vi "AB_820_850_Project_DestinationItems.vi"(6 "usedDestinations":i32[](array[numeric]), 7 "action":T3, 8 "error in (no error)":errorcluster, 9 "buildType":T1, 10 "oldBuildObject":T2, 11 "buildObject":T2) -> (0 "error out":errorcluster, 3 "buildObject out":T2)   [LabVIEW 2020]
doc: "Reads and writes the data to the object property bag."
uses:
  <resource>/Framework/Providers/API/ItemRef.ctl
  <vilib>/AppBuilder/RW_Project/AB_RW_Project_PropBag_ArrayAction.ctl
  <vilib>/AppBuilder/AB_BuildType.ctl
  <vilib>/AppBuilder/RW_Project/AB_RW_Project_PropBag_Action.ctl
  <resource>/Framework/Providers/Common/provcom_StringGlobals.vi
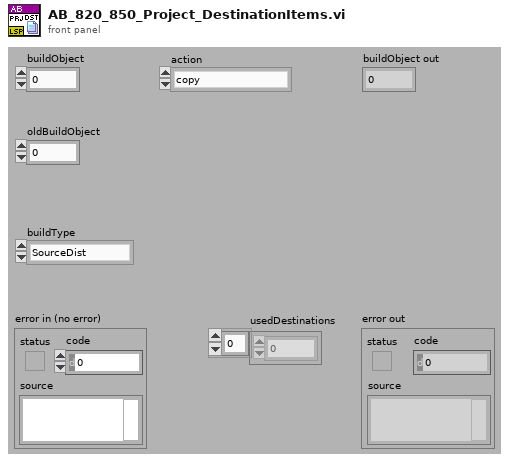
[diagram p1: front panel]
types:
  T1 = typedef "AB_BuildType.ctl" = enum16{"SourceDist", "EXE", "DLL", "RTExe"}
  T2 = typedef "ItemRef.ctl" = u64
  T3 = typedef "AB_RW_Project_PropBag_ArrayAction.ctl" = enum16{"copy", "saveForPrevious", "loadFromPrevious", "clear"}
  T4 = typedef "AB_RW_Project_PropBag_Action.ctl" = enum16{"read", "write", "clear", "readPrevious", "writePrevious", "clearPrevious"}
  T5 = cluster{"destName":string, "path":path, "preserveHierarchy":bool, "libraryName":string}
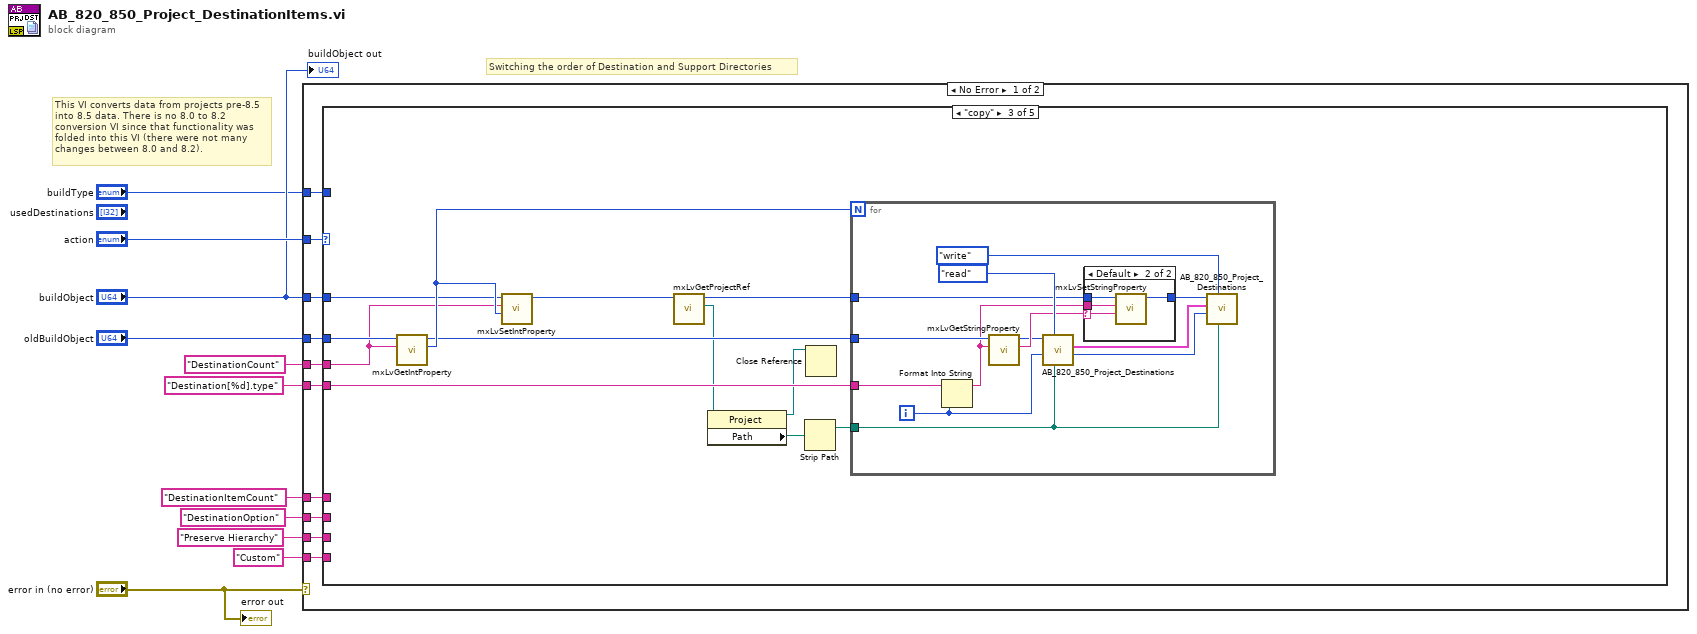
[diagram p0: block diagram]
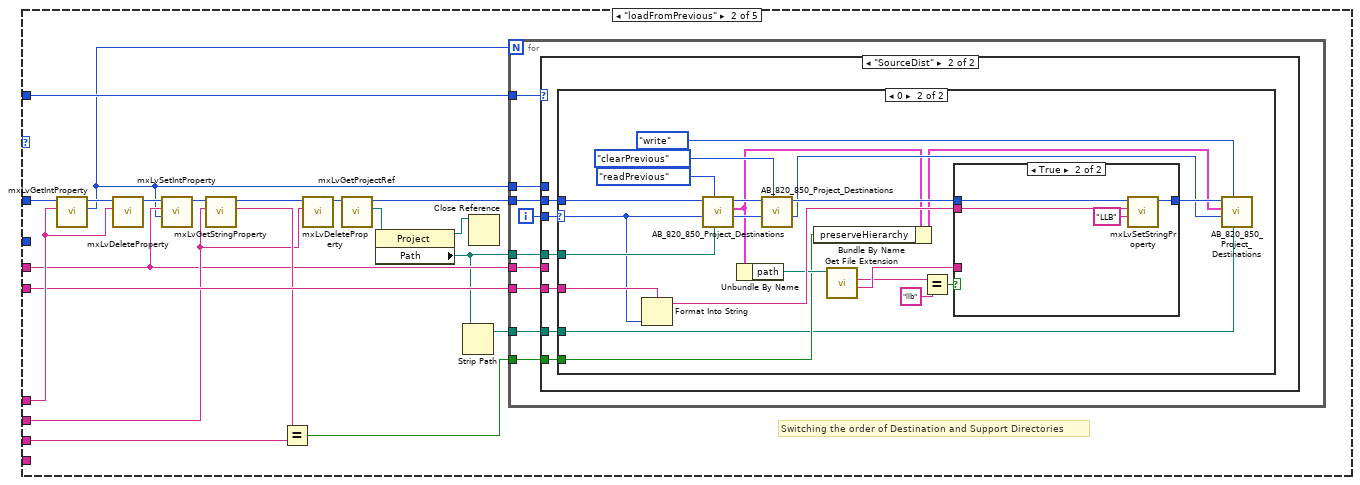
[diagram p3: hidden frame]
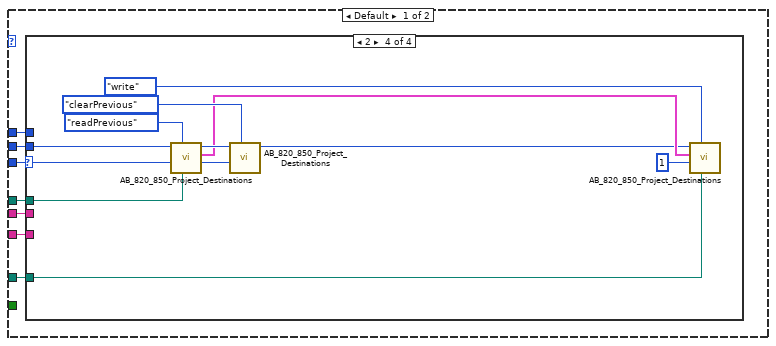
[diagram p4: hidden frame]
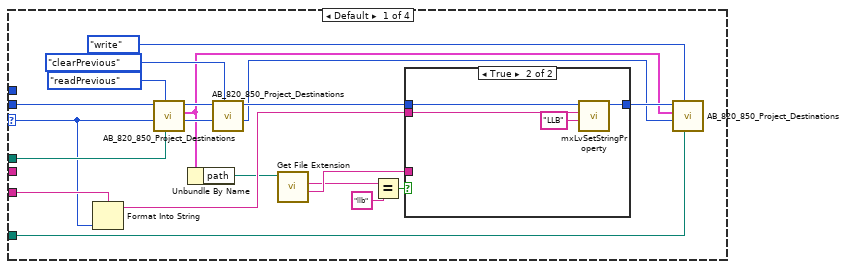
[diagram p5: hidden frame]
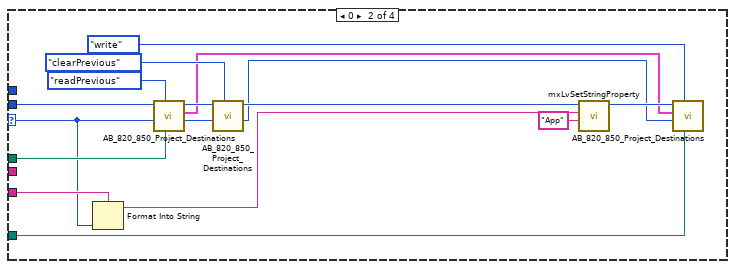
[diagram p7: hidden frame]
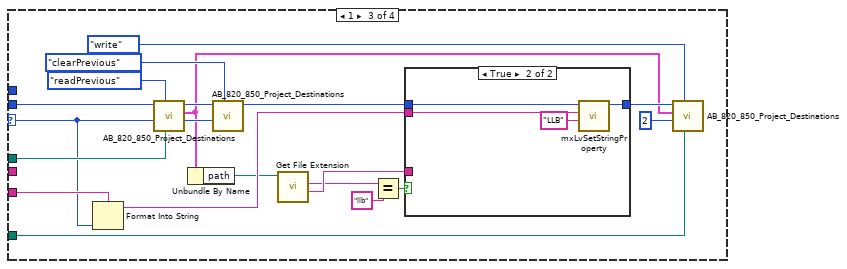
[diagram p8: hidden frame]
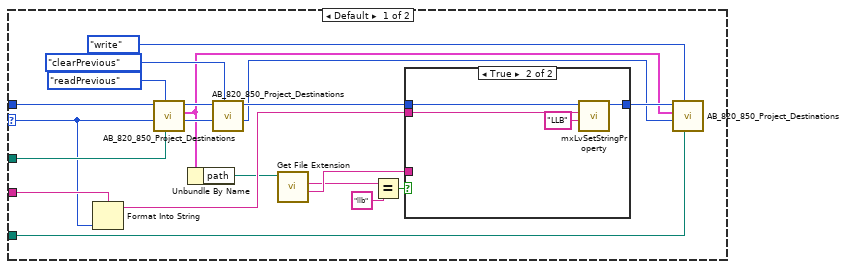
[diagram p10: hidden frame]
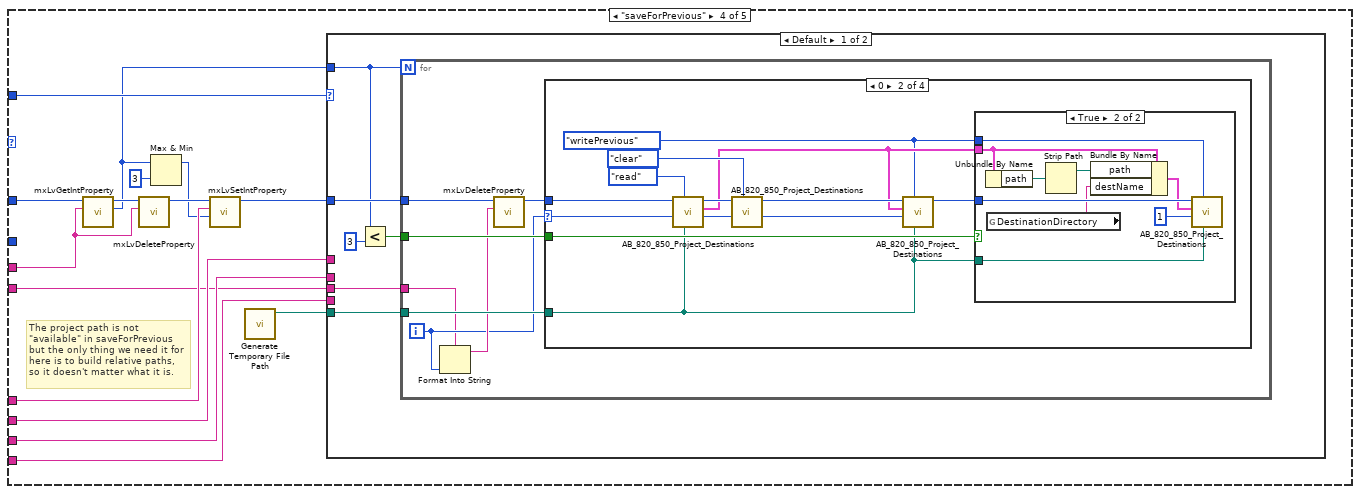
[diagram p14: hidden frame]
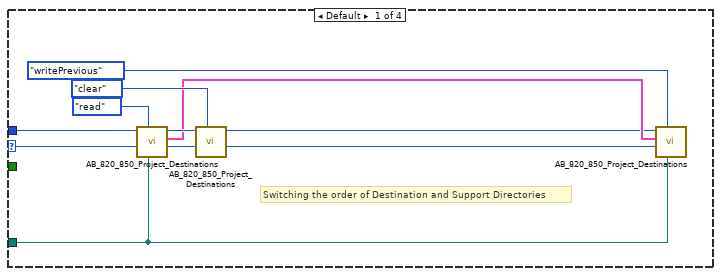
[diagram p15: hidden frame]
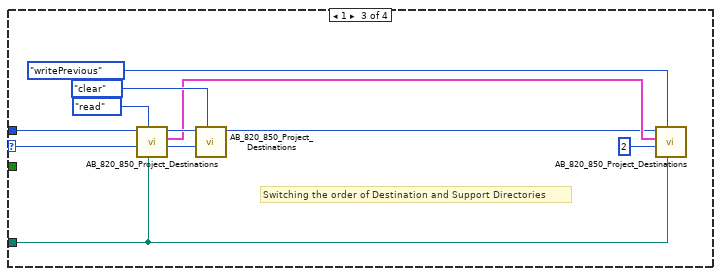
[diagram p17: hidden frame]
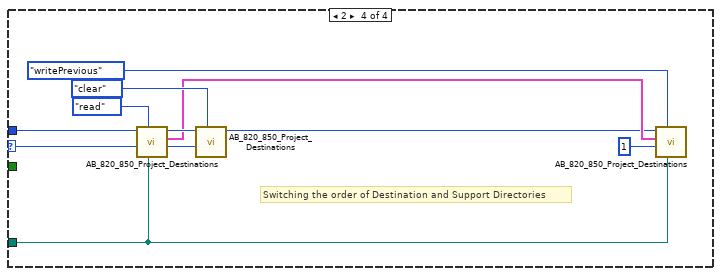
[diagram p18: hidden frame]
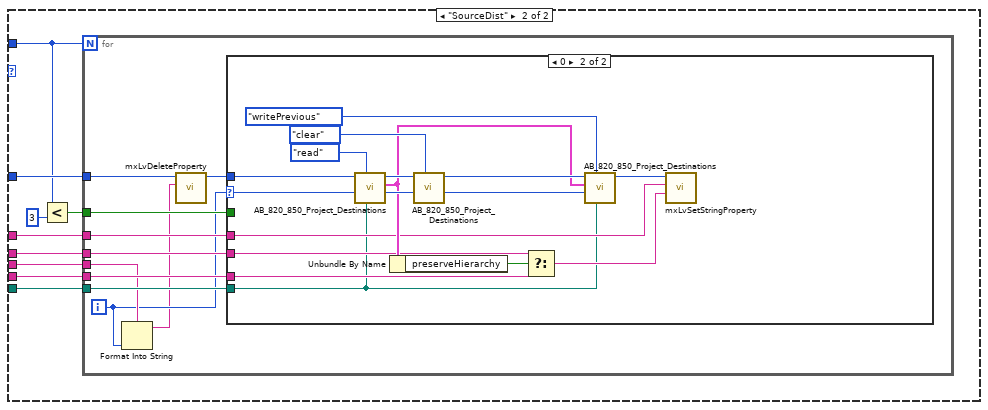
[diagram p19: hidden frame]
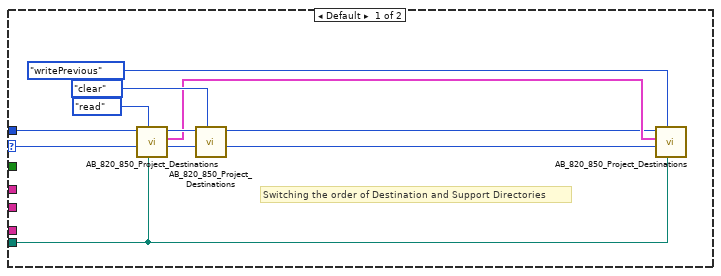
[diagram p20: hidden frame]
diagram:
  # "This VI converts data from projects pre-8.5 into 8.5 data. There is no 8.0 to 8.2 conversion VI since that functionality was folded into this VI (there were not many changes between 8.0 and 8.2)."
  # "Switching the order of Destination and Support Directories"
  n1 = case shown="No Error" "error in (no error)" {
    tunnel: "action" -> [w21 _]
    tunnel: "buildObject" -> [w20 _]
    tunnel: "DestinationCount" -> [w19 _]
    tunnel: "Destination[%d].type" -> [w18 _]
    tunnel: "DestinationItemCount" ("Tag") -> [w17 _]
    tunnel: "oldBuildObject" -> [w16 _]
    tunnel: "buildType" -> [w15 _]
    tunnel: "DestinationOption" ("Tag") -> [w14 _]
    tunnel: "Preserve Hierarchy" ("Tag") -> [w13 _]
    tunnel: "Custom" ("Tag") -> [w12 _]
    frame No Error {
      n2 = case shown="\"copy\"" w21 {
        tunnel: w20 -> [_ w41 w201 w229 w359]
        tunnel: w19 -> [_ w25 w202 w236 w356]
        tunnel: w18 -> [_ w37 w205 w227 w354]
        tunnel: w17 -> [_ w38 _ w233 _]
        tunnel: w16 -> [_ _ w203 _ _]
        tunnel: w15 -> [_ w34 _ w234 _]
        tunnel: w14 -> [_ w27 _ w232 _]
        tunnel: w13 -> [_ w31 _ w231 _]
        tunnel: w12 -> [_ _ _ w230 _]
        frame Default {
        }
        frame "loadFromPrevious" {
          # "Switching the order of Destination and Support Directories"
          n3 = call <resource>:"mxLvGetIntProperty.vi"("Tag"=w38, "Item"=w41) -> ("Value"=w24:i32, "Item"=w40:T2)  [unwired: 7 in, 1 out]
          n4 = call <resource>:"mxLvDeleteProperty.vi"("Tag"=w38, "Item"=w40) -> ("Item"=w39:T2)  [unwired: 8 in, 1 out]
          n5 = call <resource>:"mxLvSetIntProperty.vi"("Value (0)"=w24, "Tag"=w25, "Item"=w39) -> ("Item"=w33:T2)  [unwired: 7 in, 1 out]
          n6 = call <resource>:"mxLvGetStringProperty.vi"("Tag"=w27, "Item"=w33) -> ("Value"=w32:string, "Item"=w29:T2)  [unwired: 7 in, 1 out]
          n7 = Equal?(x=w32, y=w31) -> (x = y?=w30:bool)
          n8 = call <resource>:"mxLvDeleteProperty.vi"("Tag"=w27, "Item"=w29) -> ("Item"=w28:T2)  [unwired: 8 in, 1 out]
          n9 = call <resource>:"mxLvGetProjectRef.vi"("Item"=w28) -> ("Project Refnum"=w36:refnum<vi>, "Item"=w35:T2)  [unwired: 8 in, 1 out]
          n10 = property class="Project"(reference=w36) -> (reference out=w22:refnum<vi>, "Path"=w23:path)  [unwired: 1 in, 1 out]
          n11 = Strip Path(path=w23) -> (stripped path=w26:path)  [unwired: 1 out]
          n12 = Close Reference(reference=w22) -> ()  [unwired: 1 in, 1 out]
          n13 = for {
            N: w24 -> [_]
            tunnel: w35 -> [w50]
            tunnel: w37 -> [w48]
            tunnel: w23 -> [w49]
            tunnel: w34 -> [w46]
            tunnel: w30 -> [w45]
            tunnel: w26 -> [w44]
            tunnel: w25 -> [w43]
            tunnel: w24 -> [w42]
            i -> [w47]
            n14 = case shown="\"SourceDist\"" w46 {
              tunnel: w50 -> [w57 w141]
              tunnel: w49 -> [w56 w140]
              tunnel: w48 -> [w55 w139]
              tunnel: w47 -> [w54 w138]
              tunnel: w45 -> [_ w137]
              tunnel: w44 -> [w53 w136]
              tunnel: w43 -> [w52 _]
              tunnel: w42 -> [w51 _]
              frame Default {
                n15 = case shown="2" w54 {
                  selector: w54 -> [w60 w86 w115 w133]
                  tunnel: w57 -> [w77 w98 w118 w135]
                  tunnel: w56 -> [w72 w93 w117 w134]
                  tunnel: w55 -> [w69 w92 w116 _]
                  tunnel: w53 -> [w58 w83 w114 w124]
                  tunnel: w52 -> [_ _ _ _]
                  tunnel: w51 -> [_ _ _ _]
                  frame Default {
                    n16 = Format Into String(format string=w69, w60) -> (resulting string=w67:string)  [unwired: 2 in, 1 out]
                    n17 = call <vilib>:"AB_820_850_Project_Destinations.vi"("ProjectPath"=w72, "action"=AB_RW_Project_PropBag_Action."readPrevious", "index"=w60, "buildObject"=w77) -> ("index out"=w73:i32, "data out"=w64:T5, "buildObject out"=w74:T2)  [unwired: 4 in, 1 out]
                    n18 = Unbundle By Name(w64) -> ("path"=w63:path)
                    n19 = call <vilib>:"AB_820_850_Project_Destinations.vi"("action"=AB_RW_Project_PropBag_Action."clearPrevious", "index"=w73, "buildObject"=w74) -> ("index out"=w59:i32, "buildObject out"=w68:T2)  [unwired: 5 in, 2 out]
                    n20 = call <vilib>:"Get File Extension.vi"("file"=w63) -> ("filename without extension"=w62:string, "lowercase file extension"=w61:string)  [unwired: 6 in, 3 out]
                    n21 = Equal?(x=w61, y="llb") -> (x = y?=w70:bool)
                    n22 = case shown="True" w70 {
                      tunnel: w62 -> [_ _]
                      tunnel: w68 -> [w78 w82]
                      tunnel: w67 -> [_ w81]
                      tunnel: [w78 w80] -> w66
                      frame False {
                      }
                      frame True {
                        n23 = call <resource>:"mxLvSetStringProperty.vi"("Value (\"\")"="LLB" ("y"), "Tag"=w81, "Item"=w82) -> ("Item"=w80:T2)  [unwired: 7 in, 1 out]
                      }
                    }
                    n24 = call <vilib>:"AB_820_850_Project_Destinations.vi"("ProjectPath"=w58, "action"=AB_RW_Project_PropBag_Action."write", "index"=w59, "data in"=w64, "buildObject"=w66) -> ()  [unwired: 3 in, 4 out]
                  }
                  frame 0 {
                    n25 = Format Into String(format string=w92, w86) -> (resulting string=w90:string)  [unwired: 2 in, 1 out]
                    n26 = call <vilib>:"AB_820_850_Project_Destinations.vi"("ProjectPath"=w93, "action"=AB_RW_Project_PropBag_Action."readPrevious", "index"=w86, "buildObject"=w98) -> ("index out"=w94:i32, "data out"=w87:T5, "buildObject out"=w95:T2)  [unwired: 4 in, 1 out]
                    n27 = call <vilib>:"AB_820_850_Project_Destinations.vi"("action"=AB_RW_Project_PropBag_Action."clearPrevious", "index"=w94, "buildObject"=w95) -> ("index out"=w85:i32, "buildObject out"=w91:T2)  [unwired: 5 in, 2 out]
                    n28 = call <resource>:"mxLvSetStringProperty.vi"("Value (\"\")"="App" ("y"), "Tag"=w90, "Item"=w91) -> ("Item"=w89:T2)  [unwired: 7 in, 1 out]
                    n29 = call <vilib>:"AB_820_850_Project_Destinations.vi"("ProjectPath"=w83, "action"=AB_RW_Project_PropBag_Action."write", "index"=w85, "data in"=w87, "buildObject"=w89) -> ()  [unwired: 3 in, 4 out]
                  }
                  frame 1 {
                    n30 = Format Into String(format string=w116, w115) -> (resulting string=w106:string)  [unwired: 2 in, 1 out]
                    n31 = call <vilib>:"AB_820_850_Project_Destinations.vi"("ProjectPath"=w117, "action"=AB_RW_Project_PropBag_Action."readPrevious", "index"=w115, "buildObject"=w118) -> ("index out"=w110:i32, "data out"=w103:T5, "buildObject out"=w111:T2)  [unwired: 4 in, 1 out]
                    n32 = Unbundle By Name(w103) -> ("path"=w102:path)
                    n33 = call <vilib>:"AB_820_850_Project_Destinations.vi"("action"=AB_RW_Project_PropBag_Action."clearPrevious", "index"=w110, "buildObject"=w111) -> ("buildObject out"=w107:T2)  [unwired: 5 in, 3 out]
                    n34 = call <vilib>:"Get File Extension.vi"("file"=w102) -> ("filename without extension"=w101:string, "lowercase file extension"=w100:string)  [unwired: 6 in, 3 out]
                    n35 = Equal?(x=w100, y="llb") -> (x = y?=w108:bool)
                    n36 = case shown="True" w108 {
                      tunnel: w101 -> [_ _]
                      tunnel: w107 -> [w119 w123]
                      tunnel: w106 -> [_ w122]
                      tunnel: [w119 w121] -> w105
                      frame False {
                      }
                      frame True {
                        n37 = call <resource>:"mxLvSetStringProperty.vi"("Value (\"\")"="LLB" ("y"), "Tag"=w122, "Item"=w123) -> ("Item"=w121:T2)  [unwired: 7 in, 1 out]
                      }
                    }
                    n38 = call <vilib>:"AB_820_850_Project_Destinations.vi"("ProjectPath"=w114, "action"=AB_RW_Project_PropBag_Action."write", "index"=2, "data in"=w103, "buildObject"=w105) -> ()  [unwired: 3 in, 4 out]
                  }
                  frame 2 {
                    n39 = call <vilib>:"AB_820_850_Project_Destinations.vi"("ProjectPath"=w134, "action"=AB_RW_Project_PropBag_Action."readPrevious", "index"=w133, "buildObject"=w135) -> ("index out"=w129:i32, "data out"=w127:T5, "buildObject out"=w130:T2)  [unwired: 4 in, 1 out]
                    n40 = call <vilib>:"AB_820_850_Project_Destinations.vi"("action"=AB_RW_Project_PropBag_Action."clearPrevious", "index"=w129, "buildObject"=w130) -> ("buildObject out"=w125:T2)  [unwired: 5 in, 3 out]
                    n41 = call <vilib>:"AB_820_850_Project_Destinations.vi"("ProjectPath"=w124, "action"=AB_RW_Project_PropBag_Action."write", "index"=1, "data in"=w127, "buildObject"=w125) -> ()  [unwired: 3 in, 4 out]
                  }
                }
              }
              frame "SourceDist" {
                n42 = case shown="0" w138 {
                  selector: w138 -> [w144 w172]
                  tunnel: w141 -> [w161 w188]
                  tunnel: w140 -> [w156 w183]
                  tunnel: w139 -> [w153 w180]
                  tunnel: w137 -> [_ w168]
                  tunnel: w136 -> [w142 w167]
                  frame Default {
                    n43 = Format Into String(format string=w153, w144) -> (resulting string=w151:string)  [unwired: 2 in, 1 out]
                    n44 = call <vilib>:"AB_820_850_Project_Destinations.vi"("ProjectPath"=w156, "action"=AB_RW_Project_PropBag_Action."readPrevious", "index"=w144, "buildObject"=w161) -> ("index out"=w157:i32, "data out"=w148:T5, "buildObject out"=w158:T2)  [unwired: 4 in, 1 out]
                    n45 = Unbundle By Name(w148) -> ("path"=w147:path)
                    n46 = call <vilib>:"AB_820_850_Project_Destinations.vi"("action"=AB_RW_Project_PropBag_Action."clearPrevious", "index"=w157, "buildObject"=w158) -> ("index out"=w143:i32, "buildObject out"=w152:T2)  [unwired: 5 in, 2 out]
                    n47 = call <vilib>:"Get File Extension.vi"("file"=w147) -> ("filename without extension"=w146:string, "lowercase file extension"=w145:string)  [unwired: 6 in, 3 out]
                    n48 = Equal?(x=w145, y="llb") -> (x = y?=w154:bool)
                    n49 = case shown="True" w154 {
                      tunnel: w146 -> [_ _]
                      tunnel: w152 -> [w162 w166]
                      tunnel: w151 -> [_ w165]
                      tunnel: [w162 w164] -> w150
                      frame False {
                      }
                      frame True {
                        n50 = call <resource>:"mxLvSetStringProperty.vi"("Value (\"\")"="LLB" ("y"), "Tag"=w165, "Item"=w166) -> ("Item"=w164:T2)  [unwired: 7 in, 1 out]
                      }
                    }
                    n51 = call <vilib>:"AB_820_850_Project_Destinations.vi"("ProjectPath"=w142, "action"=AB_RW_Project_PropBag_Action."write", "index"=w143, "data in"=w148, "buildObject"=w150) -> ()  [unwired: 3 in, 4 out]
                  }
                  frame 0 {
                    n52 = Format Into String(format string=w180, w172) -> (resulting string=w178:string)  [unwired: 2 in, 1 out]
                    n53 = call <vilib>:"AB_820_850_Project_Destinations.vi"("ProjectPath"=w183, "action"=AB_RW_Project_PropBag_Action."readPrevious", "index"=w172, "buildObject"=w188) -> ("index out"=w184:i32, "data out"=w170:T5, "buildObject out"=w185:T2)  [unwired: 4 in, 1 out]
                    n54 = Unbundle By Name(w170) -> ("path"=w175:path)
                    n55 = call <vilib>:"AB_820_850_Project_Destinations.vi"("action"=AB_RW_Project_PropBag_Action."clearPrevious", "index"=w184, "buildObject"=w185) -> ("index out"=w171:i32, "buildObject out"=w179:T2)  [unwired: 5 in, 2 out]
                    n56 = Bundle By Name(cluster=w170, "preserveHierarchy"=w168) -> (w169:T5)
                    n57 = call <vilib>:"Get File Extension.vi"("file"=w175) -> ("filename without extension"=w174:string, "lowercase file extension"=w173:string)  [unwired: 6 in, 3 out]
                    n58 = Equal?(x=w173, y="llb") -> (x = y?=w181:bool)
                    n59 = case shown="True" w181 {
                      tunnel: w174 -> [_ _]
                      tunnel: w179 -> [w189 w193]
                      tunnel: w178 -> [_ w192]
                      tunnel: [w189 w191] -> w177
                      frame False {
                      }
                      frame True {
                        n60 = call <resource>:"mxLvSetStringProperty.vi"("Value (\"\")"="LLB" ("y"), "Tag"=w192, "Item"=w193) -> ("Item"=w191:T2)  [unwired: 7 in, 1 out]
                      }
                    }
                    n61 = call <vilib>:"AB_820_850_Project_Destinations.vi"("ProjectPath"=w167, "action"=AB_RW_Project_PropBag_Action."write", "index"=w171, "data in"=w169, "buildObject"=w177) -> ()  [unwired: 3 in, 4 out]
                  }
                }
              }
            }
          }
        }
        frame "copy" {
          n62 = call <resource>:"mxLvGetIntProperty.vi"("Tag"=w202, "Item"=w203) -> ("Value"=w204:i32, "Item"=w200:T2)  [unwired: 7 in, 1 out]
          n63 = call <resource>:"mxLvSetIntProperty.vi"("Value (0)"=w204, "Tag"=w202, "Item"=w201) -> ("Item"=w198:T2)  [unwired: 7 in, 1 out]
          n64 = call <resource>:"mxLvGetProjectRef.vi"("Item"=w198) -> ("Project Refnum"=w199:refnum<vi>, "Item"=w197:T2)  [unwired: 8 in, 1 out]
          n65 = property class="Project"(reference=w199) -> (reference out=w194:refnum<vi>, "Path"=w196:path)  [unwired: 1 in, 1 out]
          n66 = Strip Path(path=w196) -> (stripped path=w195:path)  [unwired: 1 out]
          n67 = Close Reference(reference=w194) -> ()  [unwired: 1 in, 1 out]
          n68 = for {
            N: w204 -> [_]
            tunnel: w197 -> [w211]
            tunnel: w205 -> [w217]
            tunnel: w200 -> [w214]
            tunnel: w195 -> [w206]
            i -> [w207]
            n69 = Format Into String(format string=w217, w207) -> (resulting string=w213:string)  [unwired: 2 in, 1 out]
            n70 = call <resource>:"mxLvGetStringProperty.vi"("Tag"=w213, "Item"=w214) -> ("Value"=w212:string, "Item"=w210:T2)  [unwired: 7 in, 1 out]
            n71 = call <vilib>:"AB_820_850_Project_Destinations.vi"("ProjectPath"=w206, "action"=AB_RW_Project_PropBag_Action."read", "index"=w207, "buildObject"=w210) -> ("index out"=w208:i32, "data out"=w209:T5)  [unwired: 4 in, 2 out]
            n72 = case shown="Default" w212 {
              selector: w212 -> [_ w220]
              tunnel: w211 -> [w219 w223]
              tunnel: w213 -> [_ w222]
              tunnel: [w219 w221] -> w216
              frame "" {
              }
              frame Default {
                n73 = call <resource>:"mxLvSetStringProperty.vi"("Value (\"\")"=w220, "Tag"=w222, "Item"=w223) -> ("Item"=w221:T2)  [unwired: 7 in, 1 out]
              }
            }
            n74 = call <vilib>:"AB_820_850_Project_Destinations.vi"("ProjectPath"=w206, "action"=AB_RW_Project_PropBag_Action."write", "index"=w208, "data in"=w209, "buildObject"=w216) -> ()  [unwired: 3 in, 4 out]
          }
        }
        frame "saveForPrevious" {
          # "The project path is not \"available\" in saveForPrevious but the only thing we need it for here is to build relative paths, so it doesn't matter what it is."
          n75 = call <resource>:"mxLvGetIntProperty.vi"("Tag"=w236, "Item"=w229) -> ("Value"=w225:i32, "Item"=w238:T2)  [unwired: 7 in, 1 out]
          n76 = call <resource>:"mxLvDeleteProperty.vi"("Tag"=w236, "Item"=w238) -> ("Item"=w237:T2)  [unwired: 8 in, 1 out]
          n77 = Max & Min(x=w225, y=3) -> (max(x,y)=w226:i32)  [unwired: 1 out]
          n78 = call <resource>:"mxLvSetIntProperty.vi"("Value (0)"=w226, "Tag"=w233, "Item"=w237) -> ("Item"=w235:T2)  [unwired: 7 in, 1 out]
          n79 = call <vilib>:"Generate Temporary File Path.vi"() -> ("Unique Temporary File Path"=w228:path)  [unwired: 10 in, 1 out]
          n80 = case shown="Default" w234 {
            tunnel: w225 -> [w243 w314]
            tunnel: w235 -> [w244 w315]
            tunnel: w232 -> [_ w311]
            tunnel: w231 -> [_ w310]
            tunnel: w230 -> [_ w309]
            tunnel: w228 -> [w240 w308]
            tunnel: w227 -> [w239 w307]
            frame Default {
              n81 = Less?(x=w243, y=3) -> (x < y?=w241:bool)
              n82 = for {
                N: w243 -> [_]
                tunnel: w244 -> [w248]
                tunnel: w241 -> [w251]
                tunnel: w240 -> [w250]
                tunnel: w239 -> [w245]
                i -> [w246]
                n83 = Format Into String(format string=w245, w246) -> (resulting string=w249:string)  [unwired: 2 in, 1 out]
                n84 = call <resource>:"mxLvDeleteProperty.vi"("Tag"=w249, "Item"=w248) -> ("Item"=w247:T2)  [unwired: 8 in, 1 out]
                n85 = case shown="0" w246 {
                  selector: w246 -> [w253 w270 w287 w298]
                  tunnel: w247 -> [w262 w275 w295 w306]
                  tunnel: w251 -> [_ w264 _ _]
                  tunnel: w250 -> [w252 w263 w285 w296]
                  frame Default {
                    # "Switching the order of Destination and Support Directories"
                    n86 = call <vilib>:"AB_820_850_Project_Destinations.vi"("ProjectPath"=w252, "action"=AB_RW_Project_PropBag_Action."read", "index"=w253, "buildObject"=w262) -> ("index out"=w258:i32, "data out"=w256:T5, "buildObject out"=w259:T2)  [unwired: 4 in, 1 out]
                    n87 = call <vilib>:"AB_820_850_Project_Destinations.vi"("action"=AB_RW_Project_PropBag_Action."clear", "index"=w258, "buildObject"=w259) -> ("index out"=w254:i32, "buildObject out"=w255:T2)  [unwired: 5 in, 2 out]
                    n88 = call <vilib>:"AB_820_850_Project_Destinations.vi"("ProjectPath"=w252, "action"=AB_RW_Project_PropBag_Action."writePrevious", "index"=w254, "data in"=w256, "buildObject"=w255) -> ()  [unwired: 3 in, 4 out]
                  }
                  frame 0 {
                    w265 = AB_RW_Project_PropBag_Action."writePrevious" ("action")
                    n89 = call <vilib>:"AB_820_850_Project_Destinations.vi"("ProjectPath"=w263, "action"=AB_RW_Project_PropBag_Action."read", "index"=w270, "buildObject"=w275) -> ("index out"=w271:i32, "data out"=w266:T5, "buildObject out"=w272:T2)  [unwired: 4 in, 1 out]
                    n90 = call <vilib>:"AB_820_850_Project_Destinations.vi"("action"=AB_RW_Project_PropBag_Action."clear", "index"=w271, "buildObject"=w272) -> ("index out"=w268:i32, "buildObject out"=w269:T2)  [unwired: 5 in, 2 out]
                    n91 = call <vilib>:"AB_820_850_Project_Destinations.vi"("ProjectPath"=w263, "action"=w265, "index"=w268, "data in"=w266, "buildObject"=w269) -> ("buildObject out"=w267:T2)  [unwired: 3 in, 3 out]
                    n92 = case shown="True" w264 {
                      tunnel: w267 -> [_ w284]
                      tunnel: w266 -> [_ w278]
                      tunnel: w265 -> [_ w283]
                      tunnel: w263 -> [_ w279]
                      frame False {
                      }
                      frame True {
                        n93 = Unbundle By Name(w278) -> ("path"=w277:path)
                        n94 = global read "provcom_StringGlobals.vi" "DestinationDirectory"() -> (w280:string)
                        n95 = Strip Path(path=w277) -> (stripped path=w276:path)  [unwired: 1 out]
                        n96 = Bundle By Name(cluster=w278, "path"=w276, "destName"=w280) -> (w281:T5)
                        n97 = call <vilib>:"AB_820_850_Project_Destinations.vi"("ProjectPath"=w279, "action"=w283, "index"=1, "data in"=w281, "buildObject"=w284) -> ()  [unwired: 3 in, 4 out]
                      }
                    }
                  }
                  frame 1 {
                    # "Switching the order of Destination and Support Directories"
                    n98 = call <vilib>:"AB_820_850_Project_Destinations.vi"("ProjectPath"=w285, "action"=AB_RW_Project_PropBag_Action."read", "index"=w287, "buildObject"=w295) -> ("index out"=w291:i32, "data out"=w289:T5, "buildObject out"=w292:T2)  [unwired: 4 in, 1 out]
                    n99 = call <vilib>:"AB_820_850_Project_Destinations.vi"("action"=AB_RW_Project_PropBag_Action."clear", "index"=w291, "buildObject"=w292) -> ("buildObject out"=w288:T2)  [unwired: 5 in, 3 out]
                    n100 = call <vilib>:"AB_820_850_Project_Destinations.vi"("ProjectPath"=w285, "action"=AB_RW_Project_PropBag_Action."writePrevious", "index"=2, "data in"=w289, "buildObject"=w288) -> ()  [unwired: 3 in, 4 out]
                  }
                  frame 2 {
                    # "Switching the order of Destination and Support Directories"
                    n101 = call <vilib>:"AB_820_850_Project_Destinations.vi"("ProjectPath"=w296, "action"=AB_RW_Project_PropBag_Action."read", "index"=w298, "buildObject"=w306) -> ("index out"=w302:i32, "data out"=w300:T5, "buildObject out"=w303:T2)  [unwired: 4 in, 1 out]
                    n102 = call <vilib>:"AB_820_850_Project_Destinations.vi"("action"=AB_RW_Project_PropBag_Action."clear", "index"=w302, "buildObject"=w303) -> ("buildObject out"=w299:T2)  [unwired: 5 in, 3 out]
                    n103 = call <vilib>:"AB_820_850_Project_Destinations.vi"("ProjectPath"=w296, "action"=AB_RW_Project_PropBag_Action."writePrevious", "index"=1, "data in"=w300, "buildObject"=w299) -> ()  [unwired: 3 in, 4 out]
                  }
                }
              }
            }
            frame "SourceDist" {
              n104 = Less?(x=w314, y=3) -> (x < y?=w312:bool)
              n105 = for {
                N: w314 -> [_]
                tunnel: w315 -> [w320]
                tunnel: w312 -> [w325]
                tunnel: w311 -> [w324]
                tunnel: w310 -> [w323]
                tunnel: w309 -> [w322]
                tunnel: w308 -> [w321]
                tunnel: w307 -> [w318]
                i -> [w317]
                n106 = Format Into String(format string=w318, w317) -> (resulting string=w316:string)  [unwired: 2 in, 1 out]
                n107 = call <resource>:"mxLvDeleteProperty.vi"("Tag"=w316, "Item"=w320) -> ("Item"=w319:T2)  [unwired: 8 in, 1 out]
                n108 = case shown="0" w317 {
                  selector: w317 -> [w327 w348]
                  tunnel: w319 -> [w336 w353]
                  tunnel: w325 -> [_ _]
                  tunnel: w324 -> [_ w341]
                  tunnel: w323 -> [_ w340]
                  tunnel: w322 -> [_ w339]
                  tunnel: w321 -> [w326 w337]
                  frame Default {
                    # "Switching the order of Destination and Support Directories"
                    n109 = call <vilib>:"AB_820_850_Project_Destinations.vi"("ProjectPath"=w326, "action"=AB_RW_Project_PropBag_Action."read", "index"=w327, "buildObject"=w336) -> ("index out"=w332:i32, "data out"=w330:T5, "buildObject out"=w333:T2)  [unwired: 4 in, 1 out]
                    n110 = call <vilib>:"AB_820_850_Project_Destinations.vi"("action"=AB_RW_Project_PropBag_Action."clear", "index"=w332, "buildObject"=w333) -> ("index out"=w328:i32, "buildObject out"=w329:T2)  [unwired: 5 in, 2 out]
                    n111 = call <vilib>:"AB_820_850_Project_Destinations.vi"("ProjectPath"=w326, "action"=AB_RW_Project_PropBag_Action."writePrevious", "index"=w328, "data in"=w330, "buildObject"=w329) -> ()  [unwired: 3 in, 4 out]
                  }
                  frame 0 {
                    n112 = call <vilib>:"AB_820_850_Project_Destinations.vi"("ProjectPath"=w337, "action"=AB_RW_Project_PropBag_Action."read", "index"=w348, "buildObject"=w353) -> ("index out"=w349:i32, "data out"=w344:T5, "buildObject out"=w350:T2)  [unwired: 4 in, 1 out]
                    n113 = Unbundle By Name(w344) -> ("preserveHierarchy"=w343:bool)
                    n114 = call <vilib>:"AB_820_850_Project_Destinations.vi"("action"=AB_RW_Project_PropBag_Action."clear", "index"=w349, "buildObject"=w350) -> ("index out"=w346:i32, "buildObject out"=w347:T2)  [unwired: 5 in, 2 out]
                    n115 = Select(t=w340, s=w343, f=w339) -> (s? t:f=w338:string)
                    n116 = call <vilib>:"AB_820_850_Project_Destinations.vi"("ProjectPath"=w337, "action"=AB_RW_Project_PropBag_Action."writePrevious", "index"=w346, "data in"=w344, "buildObject"=w347) -> ("buildObject out"=w342:T2)  [unwired: 3 in, 3 out]
                    n117 = call <resource>:"mxLvSetStringProperty.vi"("Value (\"\")"=w338, "Tag"=w341, "Item"=w342) -> ()  [unwired: 7 in, 2 out]
                  }
                }
              }
            }
          }
        }
        frame "clear" {
          n118 = call <resource>:"mxLvGetIntProperty.vi"("Tag"=w356, "Item"=w359) -> ("Value"=w357:i32, "Item"=w358:T2)  [unwired: 7 in, 1 out]
          n119 = call <resource>:"mxLvDeleteProperty.vi"("Tag"=w356, "Item"=w358) -> ("Item"=w355:T2)  [unwired: 8 in, 1 out]
          n120 = for {
            N: w357 -> [_]
            tunnel: w355 -> [w364]
            tunnel: w354 -> [w362]
            i -> [w361]
            n121 = Format Into String(format string=w362, w361) -> (resulting string=w360:string)  [unwired: 2 in, 1 out]
            n122 = call <resource>:"mxLvDeleteProperty.vi"("Tag"=w360, "Item"=w364) -> ("Item"=w363:T2)  [unwired: 8 in, 1 out]
            n123 = call <vilib>:"AB_820_850_Project_Destinations.vi"("action"=AB_RW_Project_PropBag_Action."clear", "index"=w361, "buildObject"=w363) -> ()  [unwired: 5 in, 4 out]
          }
        }
      }
    }
    frame Error {
    }
  }
  "error out" <- "error in (no error)"
  "buildObject out" <- "buildObject"
